vi "Pre Launch Init.vi"(11 "Measurment Actor in":refnum<class "Measurment Actor.lvclass">) -> (0 "error out":errorcluster, 3 "Measurment Actor out":refnum<class "Measurment Actor.lvclass">)   [LabVIEW 2019, in "Measurment Actor.lvlib" / "Measurment Actor.lvclass"]
doc: "(<B>Filename</B>: Actor Framework.lvlib:Actor.lvclass:Pre Launch Init.vi)\n\nDefines behavior that occurs after the Launch Nested Actor method is invoked but before the actor's Actor Core method begins running.\n\nBy default, this method does nothing. A descendant class may override it to define behavior."
uses:
  Measurment Actor.lvclass
  Measurment Actor.lvclass/Measurment Actor.ctl
  <vilib>/ActorFramework/Actor/Actor.lvclass
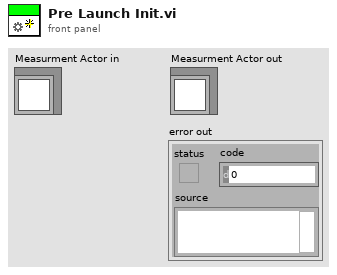
[diagram p1: front panel]
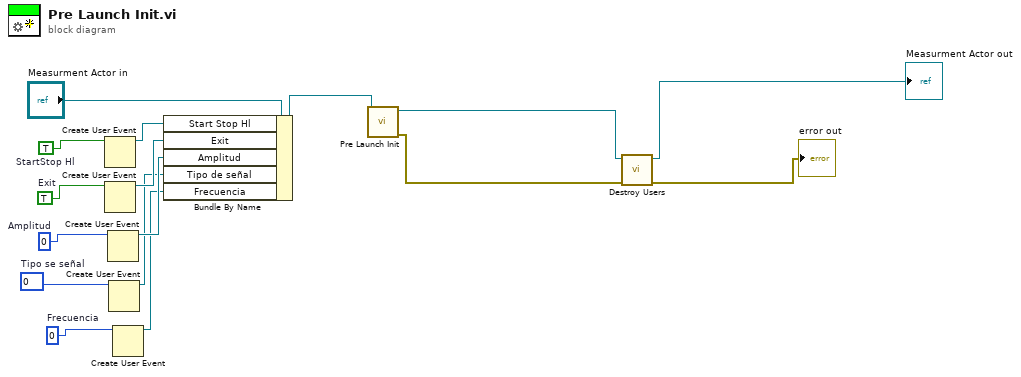
[diagram p0: block diagram]
diagram:
  w2 = u16 0 items=[""]  # Tipo se señal
  w4 = 0  # Frecuencia
  w6 = 0  # Amplitud
  w15 = TRUE  # Exit
  w14 = TRUE  # StartStop Hl
  n1 = Create User Event(user event datatype=w14) -> (user event=w12:refnum<user-event>)  [unwired: 1 in, 1 out]
  n2 = Create User Event(user event datatype=w15) -> (user event=w11:refnum<user-event>)  [unwired: 1 in, 1 out]
  n3 = Create User Event(user event datatype=w6) -> (user event=w5:refnum<user-event>)  [unwired: 1 in, 1 out]
  n4 = Create User Event(user event datatype=w2) -> (user event=w1:refnum<user-event>)  [unwired: 1 in, 1 out]
  n5 = Create User Event(user event datatype=w4) -> (user event=w3:refnum<user-event>)  [unwired: 1 in, 1 out]
  n6 = Bundle By Name(cluster="Measurment Actor in", "Start Stop Hl"=w12, "Exit"=w11, "Amplitud"=w5, "Tipo de señal"=w1, "Frecuencia"=w3) -> (w13:refnum<class "Measurment Actor.lvclass">)
  n7 = call-parent "Pre Launch Init.vi"("Actor in"=w13) -> ("error out"=w10:errorcluster, "Actor out"=w8:refnum<class "Measurment Actor.lvclass">)  [unwired: 9 in]
  n8 = call "Destroy Users.vi"("error in (no error)"=w10, "Measurment Actor in"=w8) -> ("error out"=→"error out":errorcluster, "Measurment Actor out"=→"Measurment Actor out":refnum<class "Measurment Actor.lvclass">)  [unwired: 8 in]
